vi "Kenan_Has_170519012.vi"() -> ()   [LabVIEW 2021]
uses:
  <vilib>/smtpClient/Set Message Text.vi
  <vilib>/smtpClient/LabVIEWSMTPClient.lvlib
panel:
  out "ACİL_DURUM":bool
  out "UYGUN":bool
  in  "GÖNDEREN":string
  in  "ŞİFRE":string
  in  "GÖNDERİLEN":string[](array[string])
  in  "KONU:":string
  in  "MESAJ:":string
  in  "STOP":bool
  in  "byte count":u32
  out "ANALOG_HIZ_GÖSTERGE":dbl(knob) scale=0.0..100.0
  out "DİJİTAL_HIZ_GÖSTERGE":string
  out "return count":u32
  in  "PORT SEÇİMİ":refnum<visa-resource-name>
  # "GÜVENLİK SİSTEMİ"
  # "MAIL_BİLGİLENDİRME"
  # "BİLGİ_EKRANI"
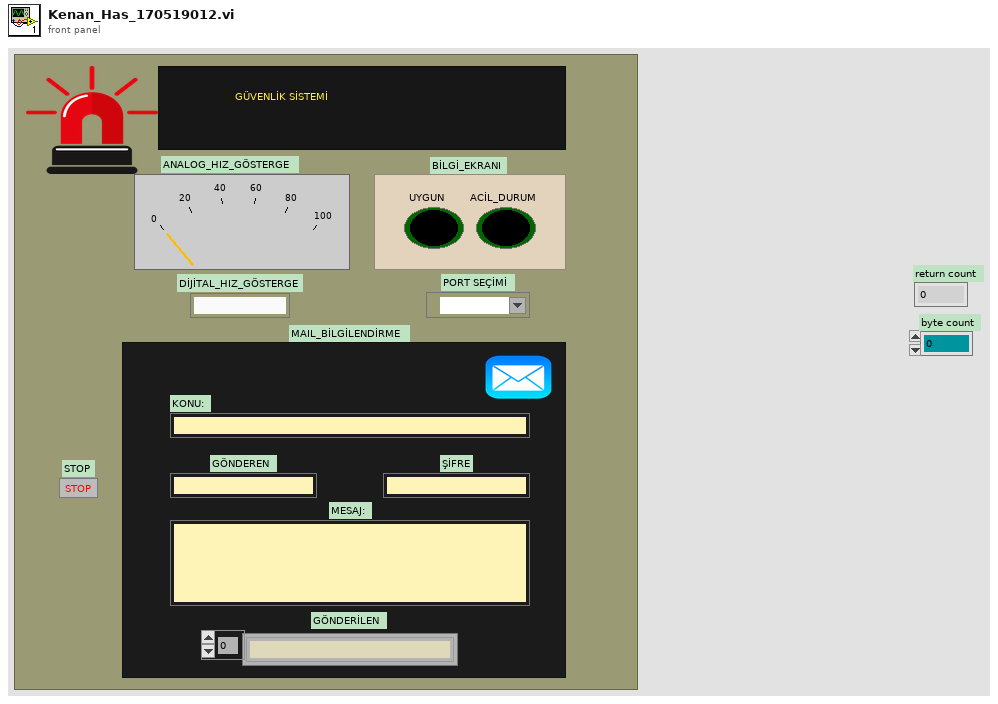
[diagram p1: front panel]
types:
  T1 = typedef "LabVIEWSMTPClient.lvlib/SmtpClientHandle.ctl" = refnum<k1>
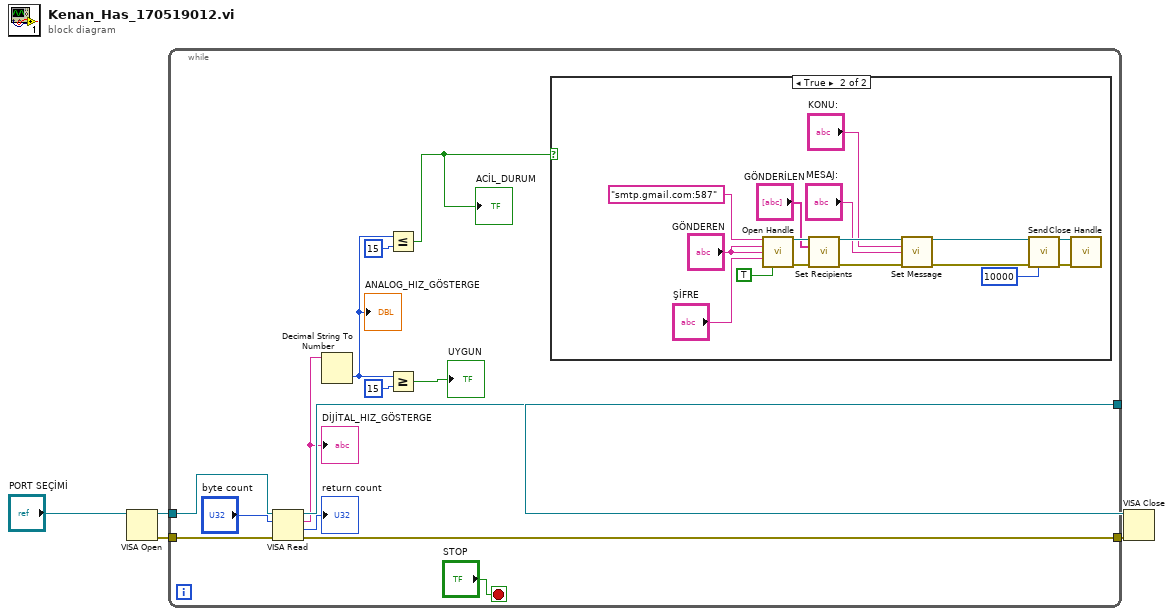
[diagram p0: block diagram]
diagram:
  n1 = VISA Open(VISA resource name="PORT SEÇİMİ") -> (VISA resource name=w4:refnum<visa-resource-name>, error out=w3:errorcluster)  [unwired: 4 in]
  n2 = while {
    tunnel: w4 -> [w17]
    tunnel: w3 -> [w15]
    tunnel: [w14] -> w2
    tunnel: [w13] -> w1
    stop <- "STOP" stop-if-true
    n3 = VISA Read(VISA resource name=w17, byte count="byte count", error in (no error)=w15) -> (VISA resource name out=w13:refnum<visa-resource-name>, read buffer=w11:string, return count=→"return count":u32, error out=w14:errorcluster)
    "DİJİTAL_HIZ_GÖSTERGE" <- w11
    n4 = Decimal String To Number(string=w11) -> (number=w10:i32)  [unwired: 2 in, 1 out]
    "ANALOG_HIZ_GÖSTERGE" <- w10
    n5 = Less Or Equal?(x=w10, y=15) -> (x <= y?=w6:bool)
    "ACİL_DURUM" <- w6
    n6 = Greater Or Equal?(x=w10, y=15) -> (x >= y?=→"UYGUN":bool)
    n7 = case shown="True" w6 {
      frame False {
      }
      frame True {
        n8 = call <vilib>:"Open Handle.vi"("server address"="smtp.gmail.com:587", "from"="GÖNDEREN", "username"="GÖNDEREN", "password"="ŞİFRE", "use TLS (false)"=TRUE) -> ("handle out"=w34:T1, "error out"=w30:errorcluster)  [unwired: 9 in]
        n9 = call <vilib>:"Set Recipients.vi"("handle in"=w34, "to"="GÖNDERİLEN", "error in (no error)"=w30) -> ("handle out"=w33:T1, "error out"=w29:errorcluster)  [unwired: 11 in]
        n10 = call-poly <vilib>:"Set Message.vi"("handle in"=w33, "subject"="KONU:", "plain text message"="MESAJ:", "error in (no error)"=w29) -> ("handle out"=w32:T1, "error out"=w28:errorcluster)  [unwired: 10 in]
        n11 = call <vilib>:"Send.vi"("handle in"=w32, "error in (no error)"=w28, "timeout in ms (10000)"=10000) -> ("handle out"=w31:T1, "error out"=w27:errorcluster)  [unwired: 10 in, 1 out]
        n12 = call <vilib>:"Close Handle.vi"("handle in"=w31, "error in (no error)"=w27) -> ()  [unwired: 12 in, 2 out]
      }
    }
  }
  n13 = VISA Close(VISA resource name=w1, error in (no error)=w2) -> ()  [unwired: 1 out]
